vi "Make Type String.vi"(8 "error in (no error)":errorcluster, 10 "Map Type":T1) -> (0 "error out":errorcluster, 2 "maptype string":string)   [LabVIEW 2012]
doc: "Creates the required zoom string."
uses:
  TypeDefs/Map Types.ctl
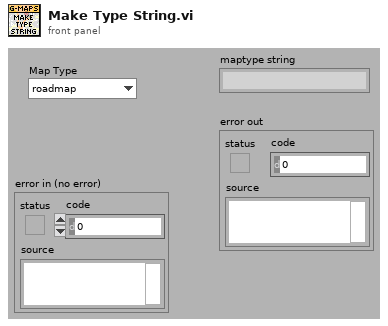
[diagram p1: front panel]
types:
  T1 = typedef "Map Types.ctl" = enum16{"roadmap", "satellite", "terrain", "hybrid"}
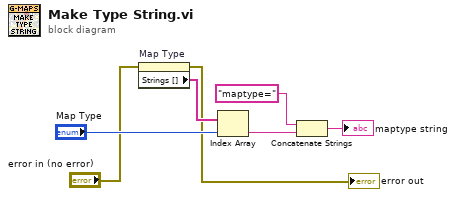
[diagram p0: block diagram]
diagram:
  n1 = property on="Map Type" class="Enum (strict)"(error in="error in (no error)") -> (error out=→"error out":errorcluster, "Strings []"=w5:string[])  [unwired: 1 in, 1 out]
  n2 = Index Array(array=w5, index="Map Type") -> (element=w3:string)
  n3 = Concatenate Strings("maptype=" ("URL"), w3) -> (→"maptype string":string)
